vi "Setcan_comm.vi"(8 "error in (no error)":errorcluster, 10 "Set_Val":T1, 11 "OneOfTemplate in":refnum<class "nixnet_grpc_ReadStateValue_value.lvclass">) -> (0 "error out":errorcluster, 3 "OneOfTemplate out":refnum<class "nixnet_grpc_ReadStateValue_value.lvclass">)   [LabVIEW 2019, in "grpc-xnet_client.lvlib" / "nixnet_grpc_ReadStateValue_value.lvclass"]
uses:
  nixnet_grpc_ReadStateValue_value.lvclass
  nixnet_grpc_CanCommResponse.ctl
  nixnet_grpc_CanCommState.ctl
  nixnet_grpc_CanLastErr.ctl
  nixnet_grpc_ReadStateValue_value.lvclass/nixnet_grpc_ReadStateValue_value.ctl
  grpc-xnet_client.lvlib
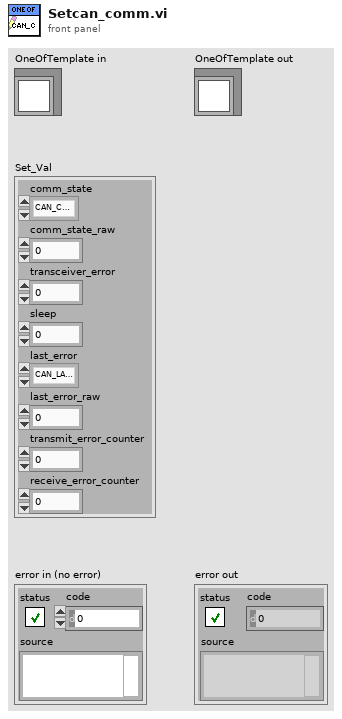
[diagram p1: front panel]
types:
  T1 = typedef "grpc-xnet_client.lvlib/nixnet_grpc_CanCommResponse.ctl" = cluster{"comm_state":T2, "comm_state_raw":u32, "transceiver_error":u32, "sleep":u32, "last_error":T3, "last_error_raw":u32, "transmit_error_counter":u32, "receive_error_counter":u32}
  T2 = typedef "grpc-xnet_client.lvlib/nixnet_grpc_CanCommState.ctl" = enum32{"CAN_COMM_STATE_ERROR_ACTIVE", "CAN_COMM_STATE_ERROR_PASSIVE", "CAN_COMM_STATE_BUS_OFF", "CAN_COMM_STATE_INIT"}
  T3 = typedef "grpc-xnet_client.lvlib/nixnet_grpc_CanLastErr.ctl" = enum32{"CAN_LAST_ERR_NONE", "CAN_LAST_ERR_STUFF", "CAN_LAST_ERR_FORM", "CAN_LAST_ERR_ACK", "CAN_LAST_ERR_BIT_1", "CAN_LAST_ERR_BIT_0", "CAN_LAST_ERR_CRC"}
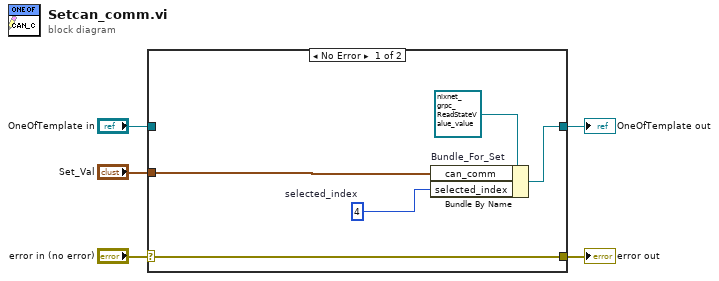
[diagram p0: block diagram]
diagram:
  n1 = case shown="No Error" "error in (no error)" {
    selector: "error in (no error)" -> [w10 w11]
    tunnel: [w10 w11] -> w4
    tunnel: [w9 w12] -> w2
    tunnel: "OneOfTemplate in" -> [_ w12]
    tunnel: "Set_Val" -> [w8 _]
    frame No Error {
      w7 = 4  # selected_index
      n2 = Bundle By Name "Bundle_For_Set"(cluster=refnum<class "nixnet_grpc_ReadStateValue_value.lvclass"> refnum ("OneOfTemplate in"), "can_comm"=w8, "selected_index"=w7) -> (w9:refnum<class "nixnet_grpc_ReadStateValue_value.lvclass">)
    }
    frame Error {
    }
  }
  "error out" <- w4
  "OneOfTemplate out" <- w2
